vi "Enqueue-Live graph data.vi"(8 "error in (no error)":errorcluster, 9 "Element to queue":T1, 10 "Logging queue element":T3={"Imaging Protocol"=enum."Live Imaging", "Number of Trials"=0, "Frame Size"=512, "# Averaged frames"=0, "Dwell time (us)"=0.0, "Index of Z-plane"=0, "Timelapse?"=FALSE, "Logging process is active"=FALSE, "Speed logging enabled"=FALSE, "tdms file ref"=refnum, "path"=path "", "Trial Number"=0, "Expected # points acquired"=FALSE, "Manually stopped"=FALSE, "Last trial"=FALSE, "Ch0 data"=[], "Ch1 data"=[], "Image Time"=[], "Continuous Time"=[], "Points acquired"={"Ch0 last trial"=0, "Ch1 last trial"=0, "All trials"=0}, "HW Timings File"=refnum} {"Frame Size" items=["100X100"=100, "128X128"=128, "200X200"=200, "256X256"=256, "512X512"=512, "1024x1024"=1024, "2048x2048"=2048]; "Dwell time (us)" format="%#.6g"}, 11 "Live graph data queue in":T7) -> (0 "error out":errorcluster, 3 "Live graph data queue":T7)   [LabVIEW 2017]
uses:
  Typedefs/Live graph data queue ref.ctl
  Live graphs queue/Typedefs/Live imaging queue element.ctl
  <vilib>/vision/Image Controls.llb/IMAQ Image.ctl
  Typedefs/Logging queue element.ctl
  Typedefs/Imaging Protocols enum.ctl
  Typedefs/Frame Size.ctl
  Typedefs/Acquired points count.ctl
  Typedefs/Read Write Enum.ctl
  Global Variables/General Globals.vi
panel:
  # "SUBROUTINE VI"
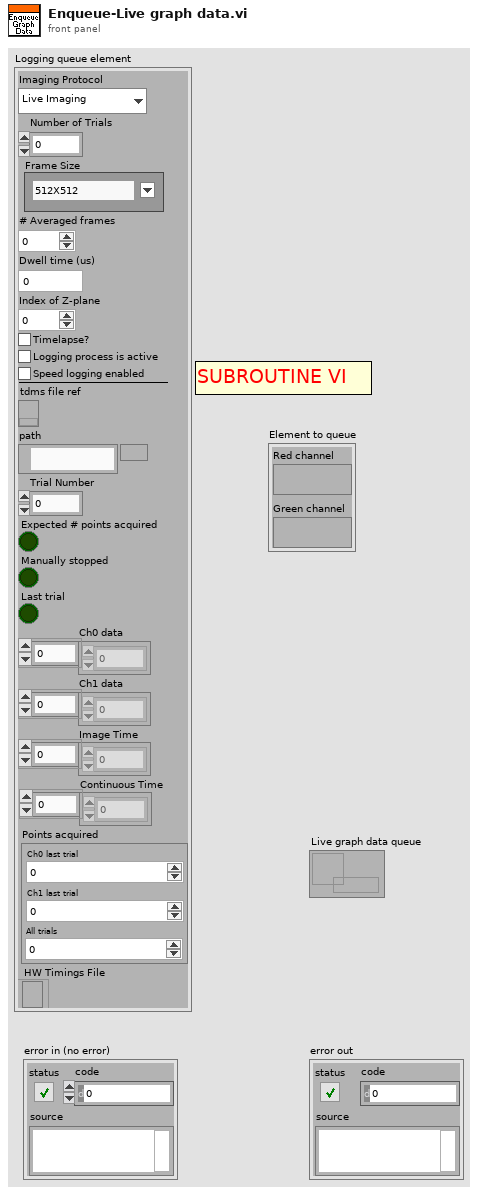
[diagram p1: front panel]
types:
  T1 = typedef "Live imaging queue element.ctl" = cluster{"Red channel":T2, "Green channel":T2}
  T2 = typedef "IMAQ Image.ctl" = refnum<image>
  T3 = typedef "Logging queue element.ctl" = cluster{"Imaging Protocol":T4, "Number of Trials":u16, "Frame Size":T5, "# Averaged frames":u16, "Dwell time (us)":dbl, "Index of Z-plane":i32, "Timelapse?":bool, "Logging process is active":bool, "Speed logging enabled":bool, "tdms file ref":refnum<k34>, "path":path, "Trial Number":i32, "Expected # points acquired":bool, "Manually stopped":bool, "Last trial":bool, "Ch0 data":u32[], "Ch1 data":u32[], "Image Time":u64[], "Continuous Time":u64[], "Points acquired":T6, "HW Timings File":refnum<file>}
  T4 = typedef "Imaging Protocols enum.ctl" = enum16{"AOL Z-Stack", "Motor Z Stack", "Functional Acquisition", "Single Plane Acquisition", "Volume Acquisition", "Live Imaging", "Live Plane Imaging", "Live Volume Imaging"}
  T5 = typedef "Frame Size.ctl" = u16
  T6 = typedef "Acquired points count.ctl" = cluster{"Ch0 last trial":u64, "Ch1 last trial":u64, "All trials":u64}
  T7 = typedef "Live graph data queue ref.ctl" = refnum<queue>
  T8 = typedef "Read Write Enum.ctl" = enum16{"Read", "Write"}
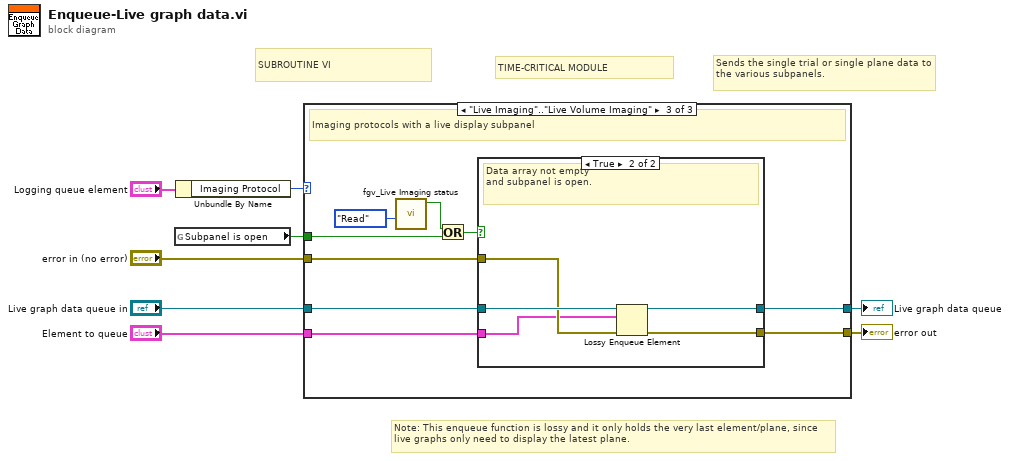
[diagram p0: block diagram]
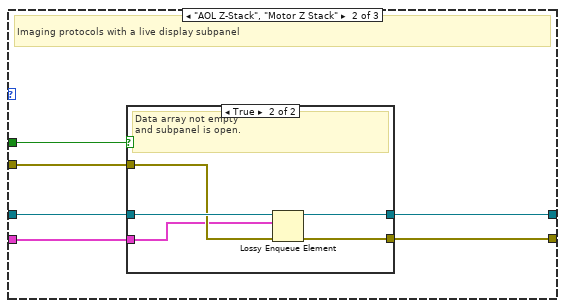
[diagram p3: hidden frame]
diagram:
  # "TIME-CRITICAL MODULE"
  # "SUBROUTINE VI"
  # "Note: This enqueue function is lossy and it only holds the very last element/plane, since live graphs only need to display the latest plane."
  # "Sends the single trial or single plane data to the various subpanels."
  n1 = global read "General Globals.vi" "Subpanel is open"() -> (w1:bool)
  n2 = Unbundle By Name("Logging queue element") -> ("Imaging Protocol"=w3:T4)
  n3 = case shown="\"Live Imaging\"..\"Live Volume Imaging\"" w3 {
    tunnel: "error in (no error)" -> [w9 w16 w32]
    tunnel: [w9 w15 w31] -> w7
    tunnel: "Live graph data queue in" -> [w10 w14 w24]
    tunnel: [w10 w13 w30] -> w5
    tunnel: "Element to queue" -> [_ w12 w29]
    tunnel: w1 -> [_ w11 w26]
    frame Default {
      # "Imaging protocols without a live display subpanel."
    }
    frame "AOL Z-Stack", "Motor Z Stack" {
      # "Imaging protocols with a live display subpanel"
      n4 = case shown="True" w11 {
        tunnel: [w17 w23] -> w15
        tunnel: [w18 w22] -> w13
        tunnel: w14 -> [w18 w21]
        tunnel: w16 -> [w17 w20]
        tunnel: w12 -> [_ w19]
        frame False {
          # "Empty data array"
        }
        frame True {
          # "Data array not empty\nand subpanel is open."
          n5 = Lossy Enqueue Element(queue=w21, element=w19, error in (no error)=w20) -> (queue out=w22:T7, error out=w23:errorcluster)  [unwired: 2 out]
        }
      }
    }
    frame "Live Imaging".."Live Volume Imaging" {
      # "Imaging protocols with a live display subpanel"
      n6 = call "fgv_Live Imaging status.vi"("Function"=Read_Write_Enum."Read") -> ("Live Imaging?"=w27:bool)  [unwired: 9 in, 1 out]
      n7 = Or(x=w27, y=w26) -> (x .or. y?=w25:bool)
      n8 = case shown="True" w25 {
        tunnel: [w33 w39] -> w31
        tunnel: [w34 w35] -> w30
        tunnel: w24 -> [w34 w38]
        tunnel: w32 -> [w33 w37]
        tunnel: w29 -> [_ w36]
        frame False {
          # "Empty data array"
        }
        frame True {
          # "Data array not empty\nand subpanel is open."
          n9 = Lossy Enqueue Element(queue=w38, element=w36, error in (no error)=w37) -> (queue out=w35:T7, error out=w39:errorcluster)  [unwired: 2 out]
        }
      }
    }
  }
  "error out" <- w7
  "Live graph data queue" <- w5
